vi "Set Value.vi"(8 "error in (no error)":errorcluster, 10 "Value":variant, 11 "Boolean Type View in":refnum<class "Boolean Type View.lvclass">) -> (0 "error out":errorcluster, 3 "Boolean Type View out":refnum<class "Boolean Type View.lvclass">)   [LabVIEW 2017, in "Boolean Type View.lvclass"]
uses:
  <vilib>/gpm_packages/@cs/Test-executive-builder/Source/Test Executive Builder Dialogs/Boolean Type View/Boolean Type View.lvclass
  <vilib>/gpm_packages/@cs/Test-executive-builder/Source/Test Executive Builder Dialogs/Boolean Type View/Boolean Type View.lvclass/Boolean Type View.ctl
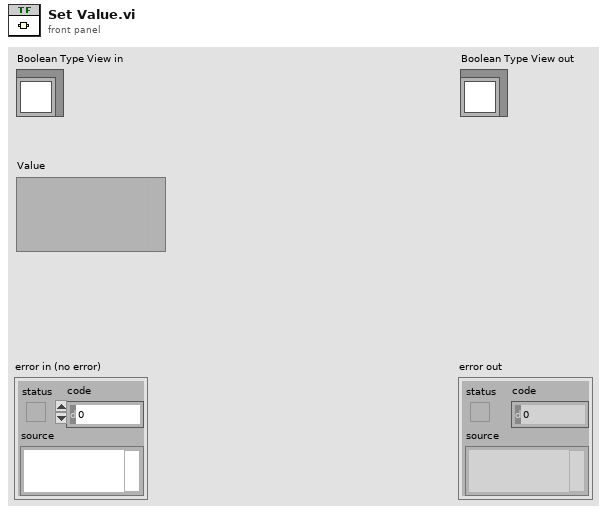
[diagram p1: front panel]
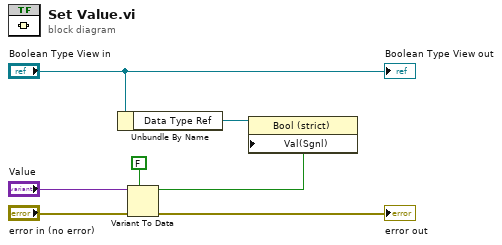
[diagram p0: block diagram]
diagram:
  n1 = Unbundle By Name("Boolean Type View in") -> ("Data Type Ref"=w7:refnum<vi>)
  n2 = Variant To Data(error in="error in (no error)", type=FALSE, Variant="Value") -> (data=w5:bool, error out=→"error out":errorcluster)
  n3 = property class="Bool (strict)"(reference=w7, "Val(Sgnl)"=w5) -> ()  [unwired: 1 in, 2 out]
  "Boolean Type View out" <- "Boolean Type View in"
